vi "FDD COOLING SS Detector Self TRAINING Ver03.vi"() -> ()   [LabVIEW 2017]
uses:
  Control 1.ctl
  <vilib>/Utility/file.llb/Read Delimited Spreadsheet (string).vi
  <vilib>/Utility/file.llb/Write Delimited Spreadsheet (string).vi
  <vilib>/Analysis/NI_AALBase.lvlib
panel:
  out "SSD LOOP Counter":i32
  out "Loop2":bool
  out "Loop1":bool
  in  "Extract \nX&Y Data?":bool
  out "DONE":bool
  in  "PAUSE?":bool
  out "% Retained":dbl format="%.1f"
  out "SS Filtered\nArray Size":i32[](array[numeric])
  out "Pre-Processed Data\nArray Size":i32[](array[numeric])
  out "Time to Execute\nSCAN (millisecond)":dbl format="%.1f"
  in  "SAVE the Conditional\nand SSD Filtered Data?":bool
  out "Selected Data\nHeader Labels":string[](array[string])
  out "Data READ LOOP Counter":i32
  out "Data Filter LOOP Counter":i32
  in  "Tab Control":T1(tab)
  out "TOTAL FILES":i32
  out "Processing File # of":i32
  out "Current File":string
  in  "READ LIST\nto PROCESS":bool
  in  "END INDEX #":i32=10
  in  "START INDEX #":i32
  in  "Renumber Dependent\nVariable INDEX Array?":bool
  in  "Output File":path=path "C:/Vance/FDD Split System Project/FY2018 Univ of Connecticut DOE FDD Project/NIST RULE BASED CHART LABVIEW FDD CODE June 2018/SS-Example_RAW_Datafile.txt"
  out "X&Y Values - Selected String Array":string[][](array[string])
  in  "Dependent Variables\nY-Values Indices":i32[](array[numeric])=[161, 162, 163, 164, 165, 166, 167, 168, 169, 170, 171, 172, 173, 174, 175, 176, 177, 178, 179, 180, 181, 182, 183, 184, 185, 186, 187, 188, 189, 190, 191, 192, 193, 194, 195, 196, 197, 198, 199, 200, 201, 202, 203, 204, 205, 206, 207, 208, 209, 210, 211, 212, 213, 214, 215, 216, 217, 218, 219, 220, 221, 222, 223, 224, 225, 226, 227, 228, 229, 230, 231, 232, 233, 234, 235, 236, 237, 238, 239, 240, 241, 242, 243, 244, 245, 246, 247, 248, 249, 250, 251, 252, 253, 254, 255, 256, 257, 258, 259, 260, 261, 262, 263, 264, 265, 266, 267, 268, 269, 270, 271, 272, 273, 274, 275, 276, 277, 278, 279, 280, 281, 282, 283, 284, 285, 286, 287, 288, 289, 290, 291, 292, 293, 294, 295, 296, 297, 298, 299, 300, 301, 302, 303, 304, 305, 306, 307, 308, 309, 310, 311, 312, 313, 314, 315, 316, 317, 318, 319, 320, 321, 322, 323, 324, 325, 326, 327, 328, 329, 330, 331, 332, 333, 334, 335, 336, 337, 338, 339, 340, 341, 342, 343, 344, 345, 346, 347, 348, 349, 350, 351, 352, 353, 354, 355, 356, 357, 358, 359, 360, 361, 362, 363, 364, 365, 366, 367, 368, 369, 370, 371, 372, 373, 374, 375, 376, 377, 378, 379, 380, 381, 382, 383, 384, 385, 386, 387, 388, 389, 390, 391, 392, 393, 394, 395, 396, 397, 398, 399, 400, 401, 402, 403, 404, 405, 406, 407, 408, 409, 410, 411, 412, 413, 414, 415, 416, 417, 418, 419, 420]
  in  "Independent Variables\nX-Values Indices":i32[](array[numeric])=[160]
  out "Input File's Header Labels":string[](array[string])=["Count", "Date", "Time", "Elapsed_Sec", "RTD#1_C", "RTD#1_Ohm", "RTD#2_C", "RTD#2_Ohm", "IEQ_Date", "IEQ_Time", "IEQ_Sec", "1100", "1101", "1102", "1103", "1104", "1105", "1106", "1107", "1108", "1109", "1110", "1111", "1112", "1113", "1114", "1115", "1200", "1201", "1202", "1203", "1204", "1205", "1206", "1207", "1208", "1209", "1210", "1211", "1212", "1213", "1214", "1215", "1300", "1301", "1302", "1303", "1304", "1305", "1306", "1307", "1308", "1309", "1310", "1311", "1312", "1313", "1314", "1315"]
  in  "Input File":path=path "C:/Vance/FDD Split System Project/FY2018 Univ of Connecticut DOE FDD Project/NIST RULE BASED CHART LABVIEW FDD CODE June 2018/Example_RAW_Datafile.txt"
  in  "Append to File (T) or\nMake NEW FILE (F)?":bool=TRUE
  out "Write Output error out":errorcluster
  in  "Delete HEADER ROW?":bool=TRUE
  in  "SELECT Array of Tests":T3(array[cluster])=[{"Selected Data - COLUMN"=8.0, "Test Function"=0, "Test Value"=500.0, "Data Label"=""}, {"Selected Data - COLUMN"=4.0, "Test Function"=2, "Test Value"=5.0, "Data Label"=""}, {"Selected Data - COLUMN"=4.0, "Test Function"=0, "Test Value"=0.0, "Data Label"=""}, {"Selected Data - COLUMN"=208.0, "Test Function"=0, "Test Value"=100.0, "Data Label"=""}, {"Selected Data - COLUMN"=63.0, "Test Function"=0, "Test Value"=100.0, "Data Label"=""}]
  out "X&Y Values - Conditional Fiiltered Data":dbl[][](array[numeric])
  out "Pre-Processed Data\nArray Size 2":i32[](array[numeric])
  out "Array of Tests w/ Labels 3":T3(array[cluster])=[{"Selected Data - COLUMN"=8.0, "Test Function"=0, "Test Value"=500.0, "Data Label"="OD_Xitron_Watts"}, {"Selected Data - COLUMN"=7.0, "Test Function"=2, "Test Value"=20.0, "Data Label"="OD_Xitron_Amps"}, {"Selected Data - COLUMN"=4.0, "Test Function"=2, "Test Value"=3.0, "Data Label"="ID_Xitron_Amps"}, {"Selected Data - COLUMN"=4.0, "Test Function"=0, "Test Value"=0.3, "Data Label"="ID_Xitron_Amps"}, {"Selected Data - COLUMN"=193.0, "Test Function"=0, "Test Value"=0.25, "Data Label"="Unit ESP (in H2O)"}, {"Selected Data - COLUMN"=193.0, "Test Function"=2, "Test Value"=0.5, "Data Label"="Unit ESP (in H2O)"}]
  out "Array of Tests w/ Labels 2":T3(array[cluster])=[{"Selected Data - COLUMN"=8.0, "Test Function"=0, "Test Value"=500.0, "Data Label"="OD_Xitron_Watts"}, {"Selected Data - COLUMN"=7.0, "Test Function"=2, "Test Value"=20.0, "Data Label"="OD_Xitron_Amps"}, {"Selected Data - COLUMN"=4.0, "Test Function"=2, "Test Value"=3.0, "Data Label"="ID_Xitron_Amps"}, {"Selected Data - COLUMN"=4.0, "Test Function"=0, "Test Value"=0.3, "Data Label"="ID_Xitron_Amps"}, {"Selected Data - COLUMN"=193.0, "Test Function"=0, "Test Value"=0.25, "Data Label"="Unit ESP (in H2O)"}, {"Selected Data - COLUMN"=193.0, "Test Function"=2, "Test Value"=0.5, "Data Label"="Unit ESP (in H2O)"}]
  out "Array of Tests w/ Labels":T3(array[cluster])=[{"Selected Data - COLUMN"=8.0, "Test Function"=0, "Test Value"=500.0, "Data Label"="OD_Xitron_Watts"}, {"Selected Data - COLUMN"=7.0, "Test Function"=2, "Test Value"=20.0, "Data Label"="OD_Xitron_Amps"}, {"Selected Data - COLUMN"=4.0, "Test Function"=2, "Test Value"=3.0, "Data Label"="ID_Xitron_Amps"}, {"Selected Data - COLUMN"=4.0, "Test Function"=0, "Test Value"=0.3, "Data Label"="ID_Xitron_Amps"}, {"Selected Data - COLUMN"=193.0, "Test Function"=0, "Test Value"=0.25, "Data Label"="Unit ESP (in H2O)"}, {"Selected Data - COLUMN"=193.0, "Test Function"=2, "Test Value"=0.5, "Data Label"="Unit ESP (in H2O)"}]
  out "XY Graph2 Label 3":string
  out "XY Graph2 Label 2":string
  out "XY Graph2 Label":string
  out "XY Graph #1 4":cluster{dbl[], dbl[]}(graph)
  in  "XY Graph1\nX-Variable 4":i32=9
  in  "XY Graph1\nY-Variable 4":i32=194
  out "XY Graph #1 3":cluster{dbl[], dbl[]}(graph)
  out "XY Graph #1 2":cluster{dbl[], dbl[]}(graph)
  in  "XY Graph1\nX-Variable 2":i32=9
  in  "XY Graph1\nY-Variable 2":i32=181
  in  "XY Graph1\nX-Variable 3":i32=9
  in  "XY Graph1\nY-Variable 3":i32=82
  out "Mean Value Y2":dbl
  out "St. Dev. Y2":dbl
  out "Mean Value Y3":dbl
  out "St. Dev. Y3":dbl
  out "Mean Value Y4":dbl
  out "St. Dev. Y4":dbl
  out "XY Graph2 Label 6":string
  out "XY Graph #1 7":cluster{dbl[], dbl[]}(graph)
  in  "XY Graph1\nX-Variable 7":i32=9
  in  "XY Graph1\nY-Variable 7":i32=218
  out "XY Graph2 Label 5":string
  out "XY Graph #1 6":cluster{dbl[], dbl[]}(graph)
  in  "XY Graph1\nX-Variable 6":i32=9
  in  "XY Graph1\nY-Variable 6":i32=91
  out "XY Graph2 Label 4":string
  out "XY Graph #1 5":cluster{dbl[], dbl[]}(graph)
  in  "XY Graph1\nX-Variable 5":i32=9
  in  "XY Graph1\nY-Variable 5":i32=4
  out "Mean Value Y5":dbl
  out "St. Dev. Y5":dbl
  out "Mean Value Y6":dbl
  out "St. Dev. Y6":dbl
  out "Mean Value Y7":dbl
  out "St. Dev. Y7":dbl
  out "XY Graph2 Label 9":string
  out "XY Graph #1 10":cluster{dbl[], dbl[]}(graph)
  in  "XY Graph1\nX-Variable 10":i32=9
  in  "XY Graph1\nY-Variable 10":i32=257
  out "Mean Value Y7 4":dbl
  out "St. Dev. Y7 4":dbl
  out "XY Graph2 Label 8":string
  out "XY Graph #1 9":cluster{dbl[], dbl[]}(graph)
  in  "XY Graph1\nX-Variable 9":i32=9
  in  "XY Graph1\nY-Variable 9":i32=205
  out "Mean Value Y7 3":dbl
  out "St. Dev. Y7 3":dbl
  out "XY Graph2 Label 7":string
  out "XY Graph #1 8":cluster{dbl[], dbl[]}(graph)
  in  "XY Graph1\nX-Variable 8":i32=9
  in  "XY Graph1\nY-Variable 8":i32=222
  out "Mean Value Y7 2":dbl
  out "St. Dev. Y7 2":dbl
  out "Steady-State Monitoring Variables 4":T4(array[cluster])=[{"Y-Value for MW"=63.0, "Y MAX Std. Deviation"=1.4, "ABS Max SLOPE"=0.004655, "X-Value for MW"=9.0}, {"Y-Value for MW"=187.0, "Y MAX Std. Deviation"=0.5, "ABS Max SLOPE"=0.00096, "X-Value for MW"=9.0}, {"Y-Value for MW"=218.0, "Y MAX Std. Deviation"=1.0, "ABS Max SLOPE"=0.0065, "X-Value for MW"=9.0}, {"Y-Value for MW"=222.0, "Y MAX Std. Deviation"=0.75, "ABS Max SLOPE"=0.0065, "X-Value for MW"=9.0}, {"Y-Value for MW"=225.0, "Y MAX Std. Deviation"=0.4, "ABS Max SLOPE"=0.004, "X-Value for MW"=9.0}, {"Y-Value for MW"=246.0, "Y MAX Std. Deviation"=0.6, "ABS Max SLOPE"=0.005, "X-Value for MW"=9.0}, {"Y-Value for MW"=181.0, "Y MAX Std. Deviation"=0.1, "ABS Max SLOPE"=1000000000.0, "X-Value for MW"=9.0}, {"Y-Value for MW"=82.0, "Y MAX Std. Deviation"=0.1, "ABS Max SLOPE"=1000000000.0, "X-Value for MW"=9.0}, {"Y-Value for MW"=194.0, "Y MAX Std. Deviation"=0.1, "ABS Max SLOPE"=1000000000.0, "X-Value for MW"=9.0}] {"ABS Max SLOPE" step=0.05; "Y MAX Std. Deviation" step=0.05 format="%_6p"}
  out "Steady-State Monitoring Variables 3":T4(array[cluster])=[{"Y-Value for MW"=63.0, "Y MAX Std. Deviation"=1.4, "ABS Max SLOPE"=0.004655, "X-Value for MW"=9.0}, {"Y-Value for MW"=187.0, "Y MAX Std. Deviation"=0.5, "ABS Max SLOPE"=0.00096, "X-Value for MW"=9.0}, {"Y-Value for MW"=218.0, "Y MAX Std. Deviation"=1.0, "ABS Max SLOPE"=0.0065, "X-Value for MW"=9.0}, {"Y-Value for MW"=222.0, "Y MAX Std. Deviation"=0.75, "ABS Max SLOPE"=0.0065, "X-Value for MW"=9.0}, {"Y-Value for MW"=225.0, "Y MAX Std. Deviation"=0.4, "ABS Max SLOPE"=0.004, "X-Value for MW"=9.0}, {"Y-Value for MW"=246.0, "Y MAX Std. Deviation"=0.6, "ABS Max SLOPE"=0.005, "X-Value for MW"=9.0}, {"Y-Value for MW"=181.0, "Y MAX Std. Deviation"=0.1, "ABS Max SLOPE"=1000000000.0, "X-Value for MW"=9.0}, {"Y-Value for MW"=82.0, "Y MAX Std. Deviation"=0.1, "ABS Max SLOPE"=1000000000.0, "X-Value for MW"=9.0}, {"Y-Value for MW"=194.0, "Y MAX Std. Deviation"=0.1, "ABS Max SLOPE"=1000000000.0, "X-Value for MW"=9.0}] {"ABS Max SLOPE" step=0.05; "Y MAX Std. Deviation" step=0.05 format="%_6p"}
  out "Steady-State Monitoring Variables 2":T4(array[cluster])=[{"Y-Value for MW"=63.0, "Y MAX Std. Deviation"=1.4, "ABS Max SLOPE"=0.004655, "X-Value for MW"=9.0}, {"Y-Value for MW"=187.0, "Y MAX Std. Deviation"=0.5, "ABS Max SLOPE"=0.00096, "X-Value for MW"=9.0}, {"Y-Value for MW"=218.0, "Y MAX Std. Deviation"=1.0, "ABS Max SLOPE"=0.0065, "X-Value for MW"=9.0}, {"Y-Value for MW"=222.0, "Y MAX Std. Deviation"=0.75, "ABS Max SLOPE"=0.0065, "X-Value for MW"=9.0}, {"Y-Value for MW"=225.0, "Y MAX Std. Deviation"=0.4, "ABS Max SLOPE"=0.004, "X-Value for MW"=9.0}, {"Y-Value for MW"=246.0, "Y MAX Std. Deviation"=0.6, "ABS Max SLOPE"=0.005, "X-Value for MW"=9.0}, {"Y-Value for MW"=181.0, "Y MAX Std. Deviation"=0.1, "ABS Max SLOPE"=1000000000.0, "X-Value for MW"=9.0}, {"Y-Value for MW"=82.0, "Y MAX Std. Deviation"=0.1, "ABS Max SLOPE"=1000000000.0, "X-Value for MW"=9.0}, {"Y-Value for MW"=194.0, "Y MAX Std. Deviation"=0.1, "ABS Max SLOPE"=1000000000.0, "X-Value for MW"=9.0}] {"ABS Max SLOPE" step=0.05; "Y MAX Std. Deviation" step=0.05 format="%_6p"}
  in  "Steady-State Monitoring Variables":T4(array[cluster])=[{"Y-Value for MW"=63.0, "Y MAX Std. Deviation"=0.5, "ABS Max SLOPE"=0.1, "X-Value for MW"=9.0}, {"Y-Value for MW"=187.0, "Y MAX Std. Deviation"=0.5, "ABS Max SLOPE"=0.1, "X-Value for MW"=9.0}, {"Y-Value for MW"=218.0, "Y MAX Std. Deviation"=0.5, "ABS Max SLOPE"=0.1, "X-Value for MW"=9.0}, {"Y-Value for MW"=222.0, "Y MAX Std. Deviation"=0.5, "ABS Max SLOPE"=0.1, "X-Value for MW"=9.0}, {"Y-Value for MW"=225.0, "Y MAX Std. Deviation"=0.5, "ABS Max SLOPE"=0.1, "X-Value for MW"=9.0}, {"Y-Value for MW"=246.0, "Y MAX Std. Deviation"=0.4, "ABS Max SLOPE"=0.1, "X-Value for MW"=9.0}, {"Y-Value for MW"=181.0, "Y MAX Std. Deviation"=0.4, "ABS Max SLOPE"=0.1, "X-Value for MW"=9.0}, {"Y-Value for MW"=82.0, "Y MAX Std. Deviation"=0.4, "ABS Max SLOPE"=0.1, "X-Value for MW"=9.0}, {"Y-Value for MW"=194.0, "Y MAX Std. Deviation"=0.4, "ABS Max SLOPE"=0.1, "X-Value for MW"=9.0}] {"ABS Max SLOPE" step=0.05; "Y MAX Std. Deviation" step=0.05 format="%_6p"}
  in  "Moving \nWindow Size":i32=22
  out "X-Variable RANGE":dbl
  out "St. Dev. Y5 6":dbl
  out "Mean Value Y5 6":dbl
  out "XY Graph SS Filtered #1":cluster{dbl[], dbl[]}(graph)
  in  "XY Graph1\nX-Variable":i32=9
  in  "XY Graph1\nY-Variable":i32=63
  out "XY Graph1 Label":string
  out "XY Graph SS Filtered #2":cluster{dbl[], dbl[]}(graph)
  in  "XY Graph2\nX-Variable 5":i32=9
  in  "XY Graph2\nY-Variable 5":i32=218
  out "XY Graph1 Label 2":string
  out "Mean Value Y":dbl
  out "St. Dev. Y":dbl
  out "XY Graph1 Label 4":string
  in  "XY Graph2\nY-Variable 7":i32=225
  in  "XY Graph2\nX-Variable 7":i32=9
  out "XY Graph SS Filtered #4":cluster{dbl[], dbl[]}(graph)
  out "Mean Value Y5 3":dbl
  out "St. Dev. Y5 3":dbl
  out "XY Graph1 Label 3":string
  in  "XY Graph2\nY-Variable 6":i32=222
  in  "XY Graph2\nX-Variable 6":i32=9
  out "XY Graph SS Filtered #3":cluster{dbl[], dbl[]}(graph)
  out "Mean Value Y5 2":dbl
  out "St. Dev. Y5 2":dbl
  out "MW Calc ERROR OUT":errorcluster
  out "XY Graph1 Label 6":string
  in  "XY Graph2\nY-Variable 9":i32=184
  in  "XY Graph2\nX-Variable 9":i32=9
  out "XY Graph SS Filtered #6":cluster{dbl[], dbl[]}(graph)
  out "Mean Value Y5 5":dbl
  out "St. Dev. Y5 5":dbl
  out "XY Graph1 Label 5":string
  in  "XY Graph2\nY-Variable 8":i32=246
  in  "XY Graph2\nX-Variable 8":i32=9
  out "XY Graph SS Filtered #5":cluster{dbl[], dbl[]}(graph)
  out "Mean Value Y5 4":dbl
  out "St. Dev. Y5 4":dbl
  out "DONE 3":bool
  out "DONE 4":bool
  out "DONE 2":bool
  # "Grab and Filter Data"
  # "Rows"
  # "Columns"
  # "Apply Conditional Filters to the Selected Data"
  # "ROWS"
  # "COLS"
  # "Conditional Filtered Data PLOTS"
  # "Conditional Filtered Data PLOTS"
  # "Conditional & SSD Filtered Data PLOTS"
  # "Display all the SS Monitoring Variables on ONE SCREEN"
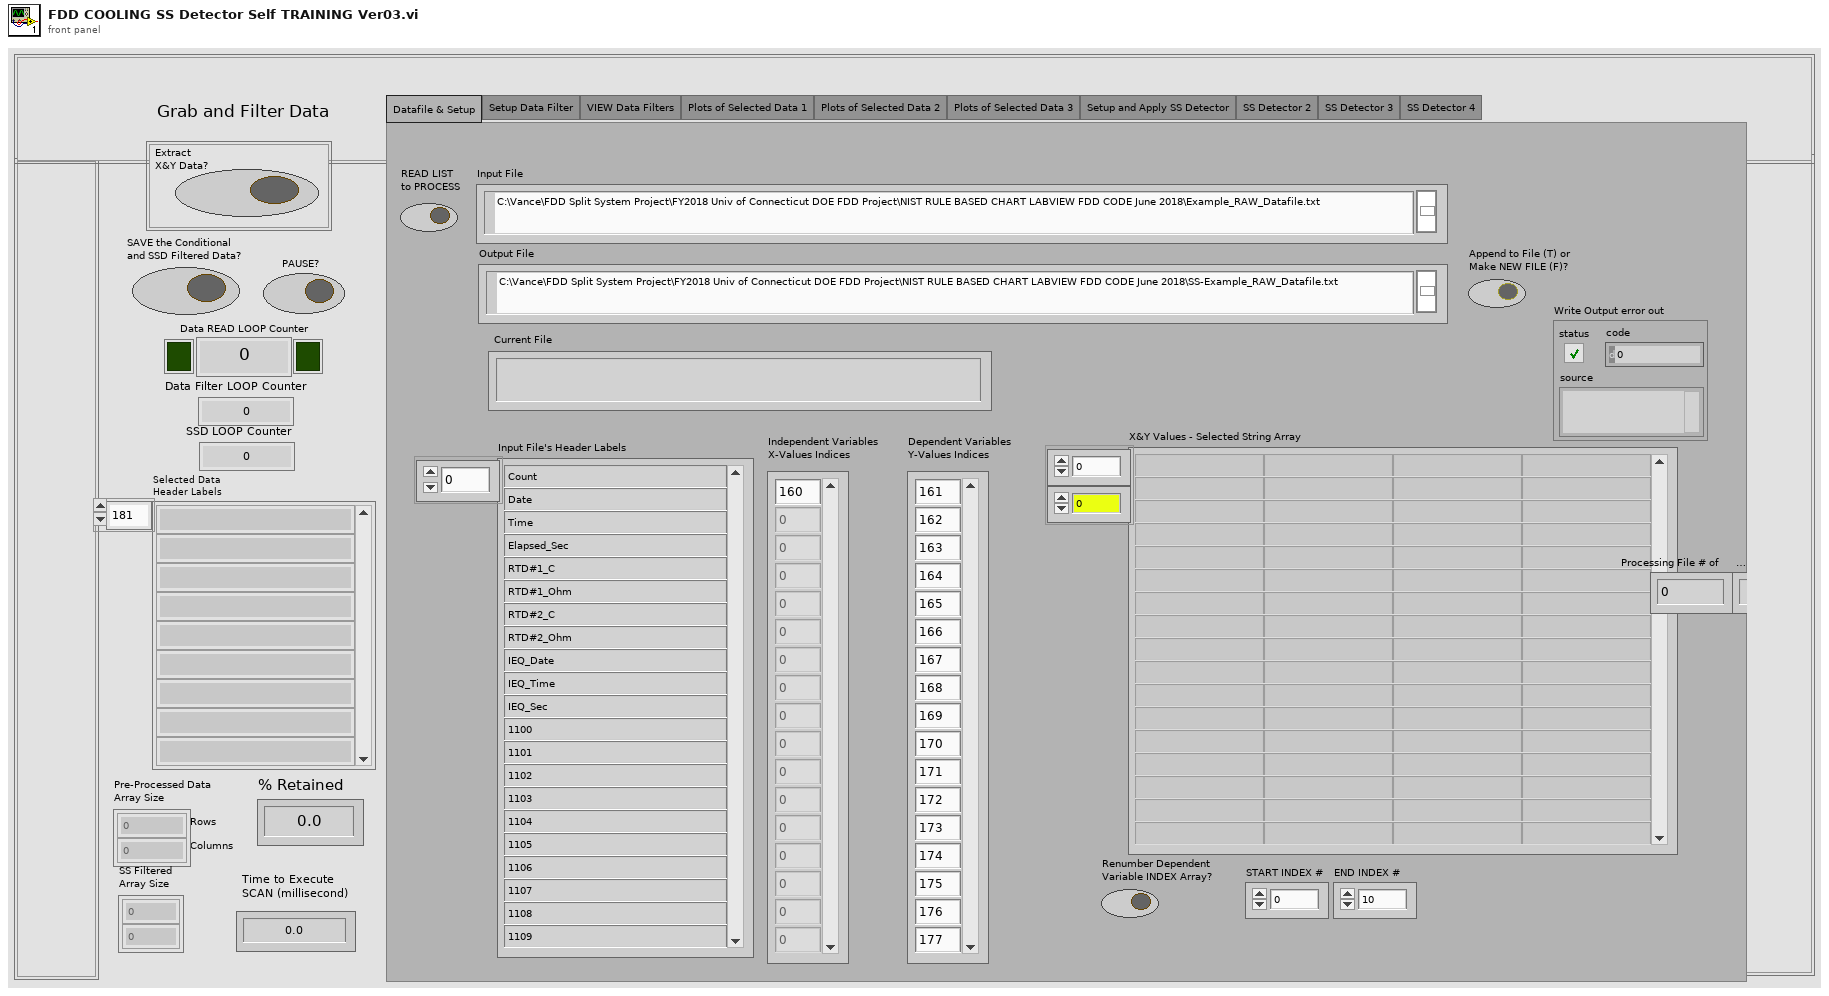
[diagram p1: front panel]
types:
  T1 = enum32{"Datafile & Setup", "Setup Data Filter", "VIEW Data Filters", "Plots of Selected Data 1", "Plots of Selected Data 2", "Plots of Selected Data 3", "Setup and Apply SS Detector", "SS Detector 2", "SS Detector 3", "SS Detector 4"}
  T2 = typedef "Control 1.ctl" = i32
  T3 = cluster{"Selected Data - COLUMN":dbl, "Test Function":T2, "Test Value":dbl, "Data Label":string}[]
  T4 = cluster{"Y-Value for MW":dbl, "Y MAX Std. Deviation":dbl, "ABS Max SLOPE":dbl, "X-Value for MW":dbl}[]
  T5 = cluster{"Selected Data - COLUMN":dbl, "Test Function":T2, "Test Value":dbl, "Data Label":string}
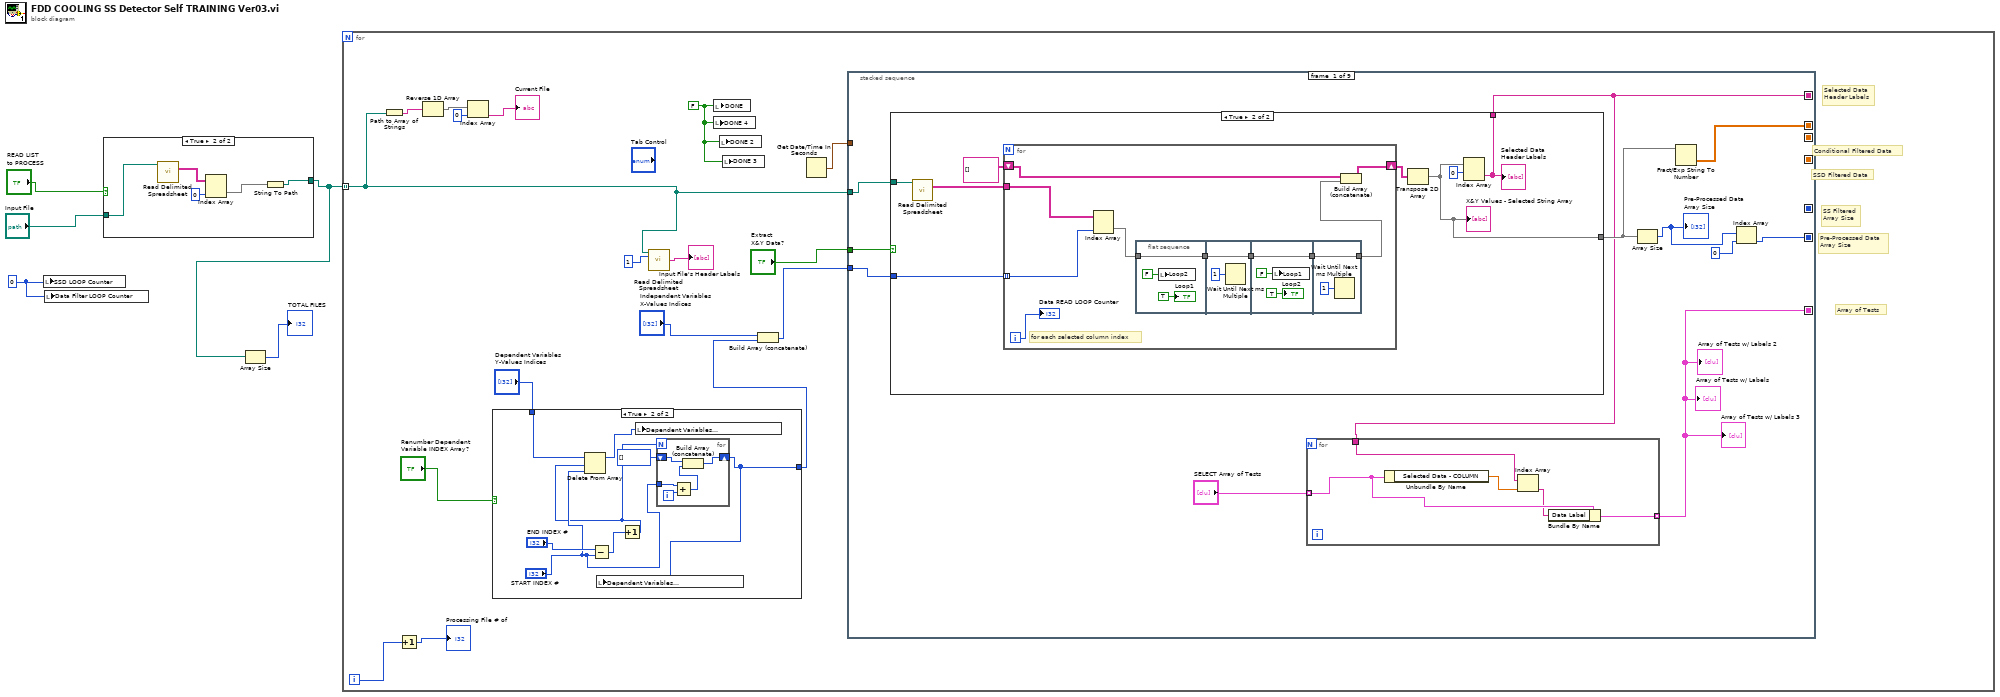
[diagram p0: block diagram]
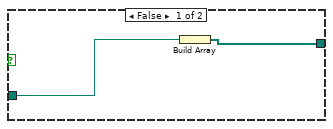
[diagram p2: hidden frame]
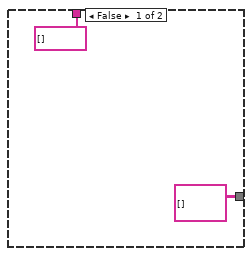
[diagram p4: hidden frame]
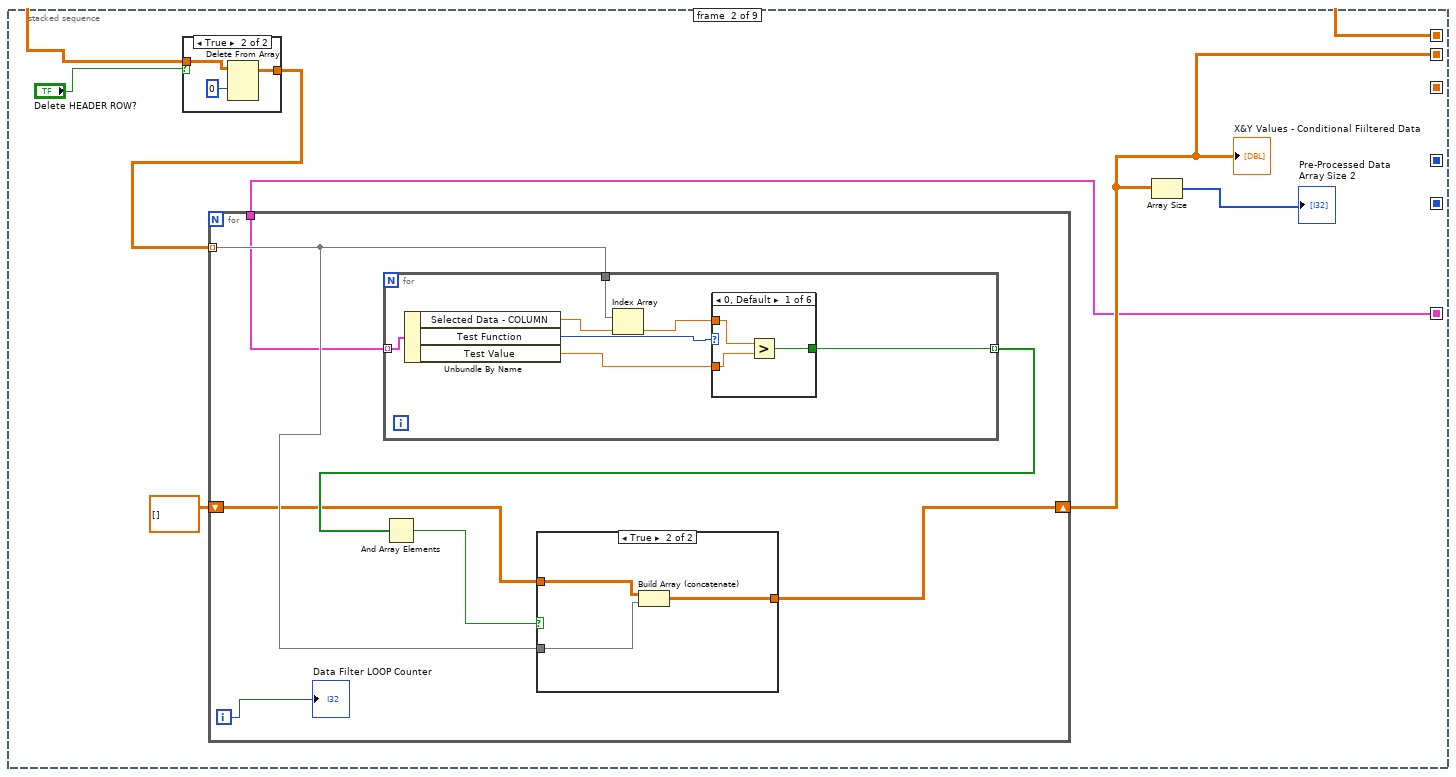
[diagram p5: hidden frame]
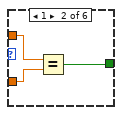
[diagram p8: hidden frame]
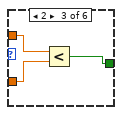
[diagram p9: hidden frame]
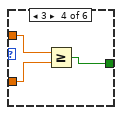
[diagram p10: hidden frame]
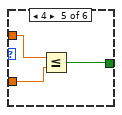
[diagram p11: hidden frame]
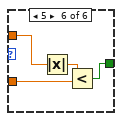
[diagram p12: hidden frame]
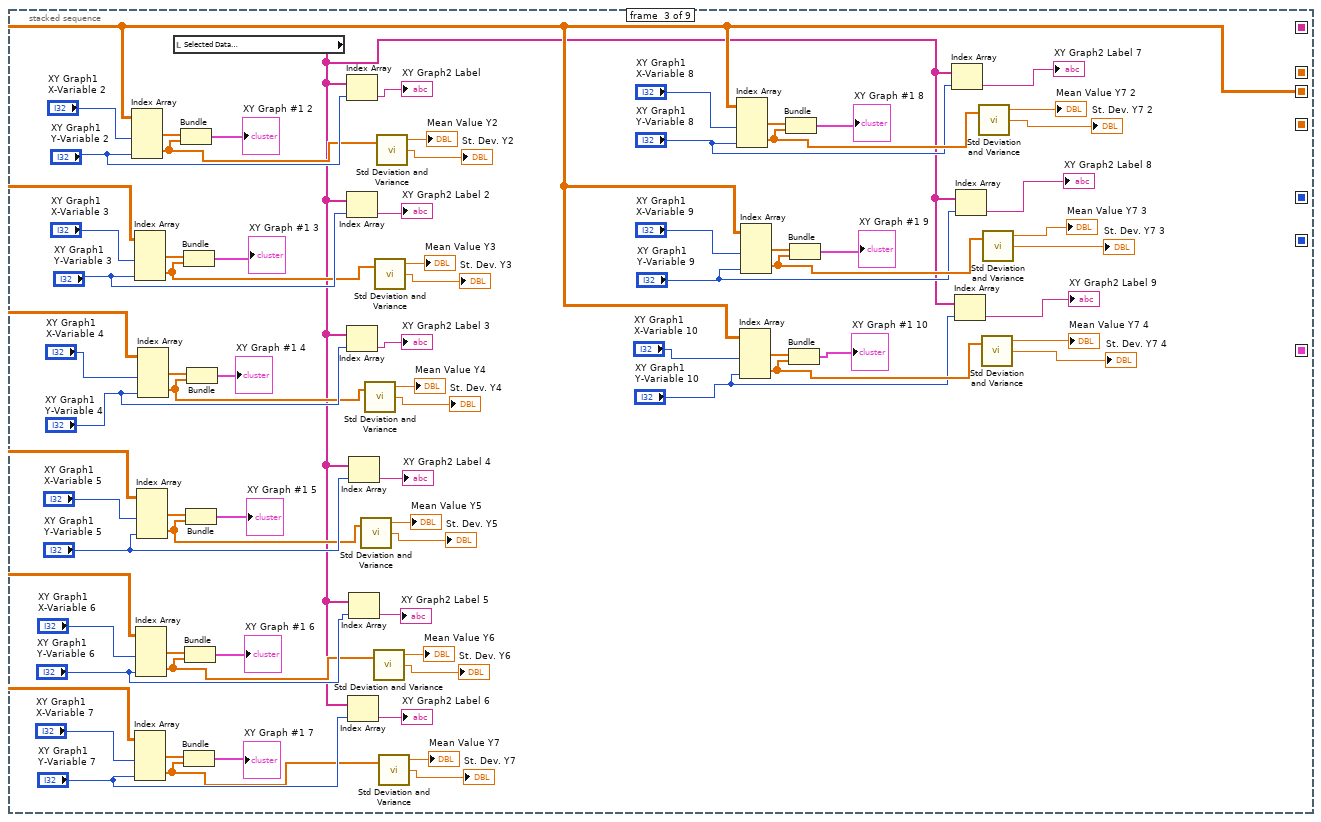
[diagram p13: hidden frame]
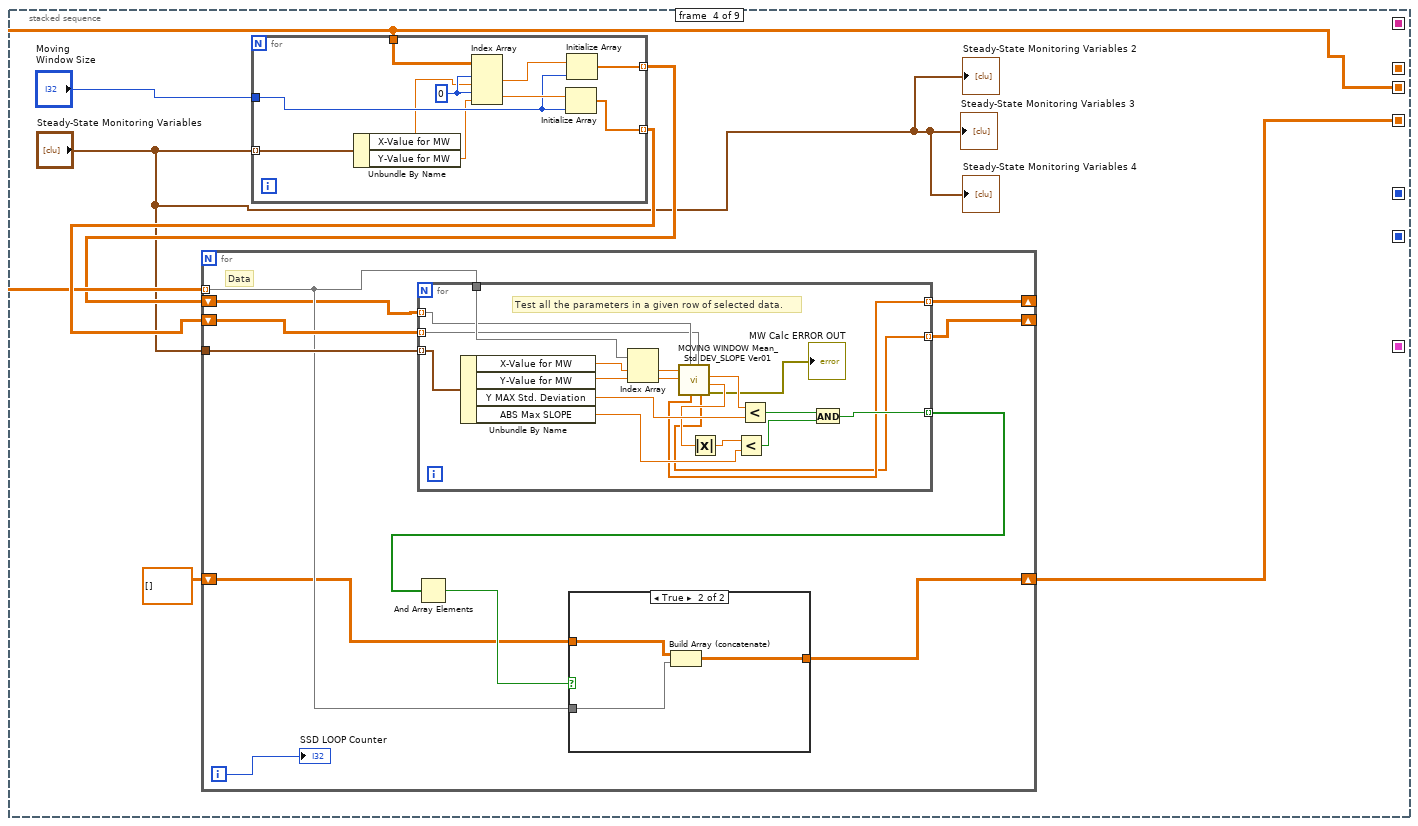
[diagram p14: hidden frame]
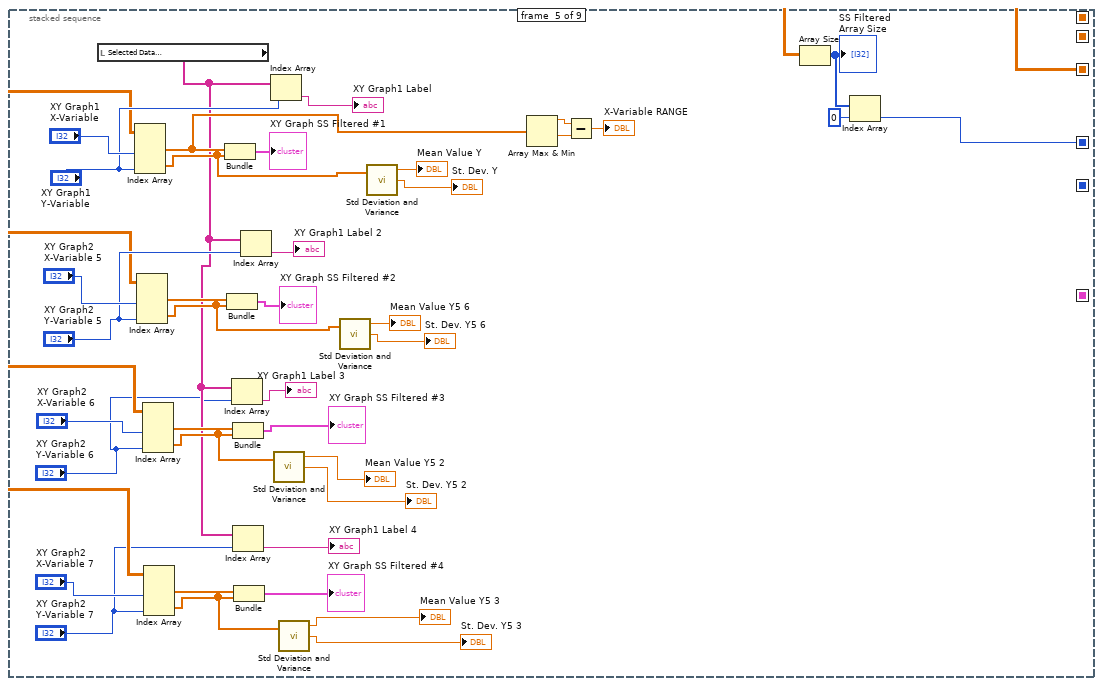
[diagram p16: hidden frame]
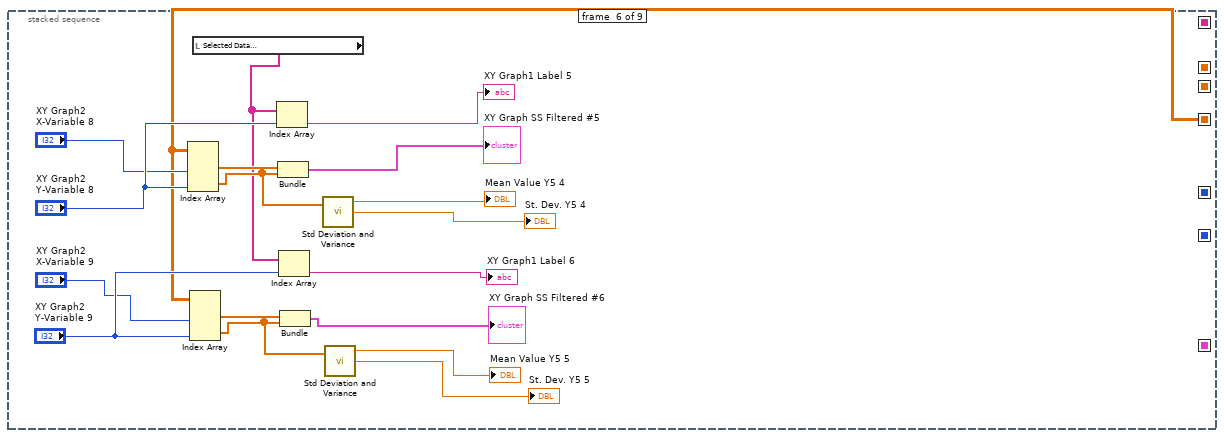
[diagram p17: hidden frame]
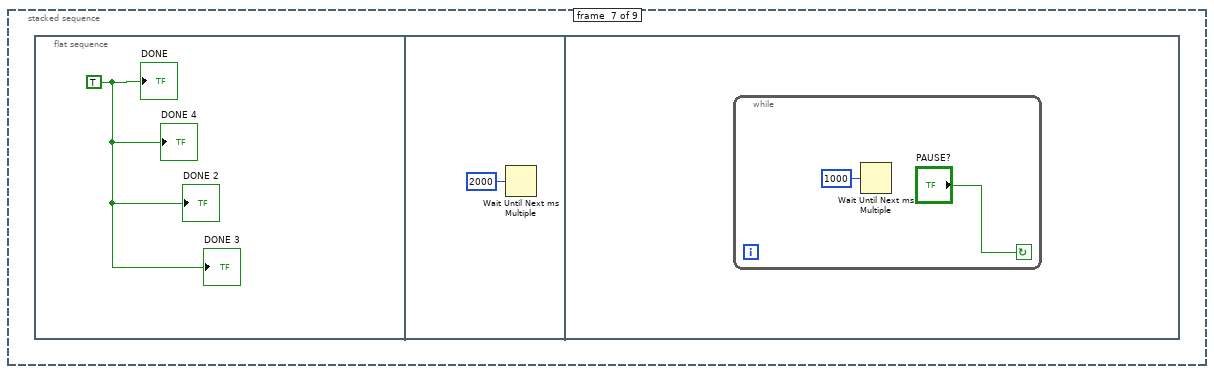
[diagram p18: hidden frame]
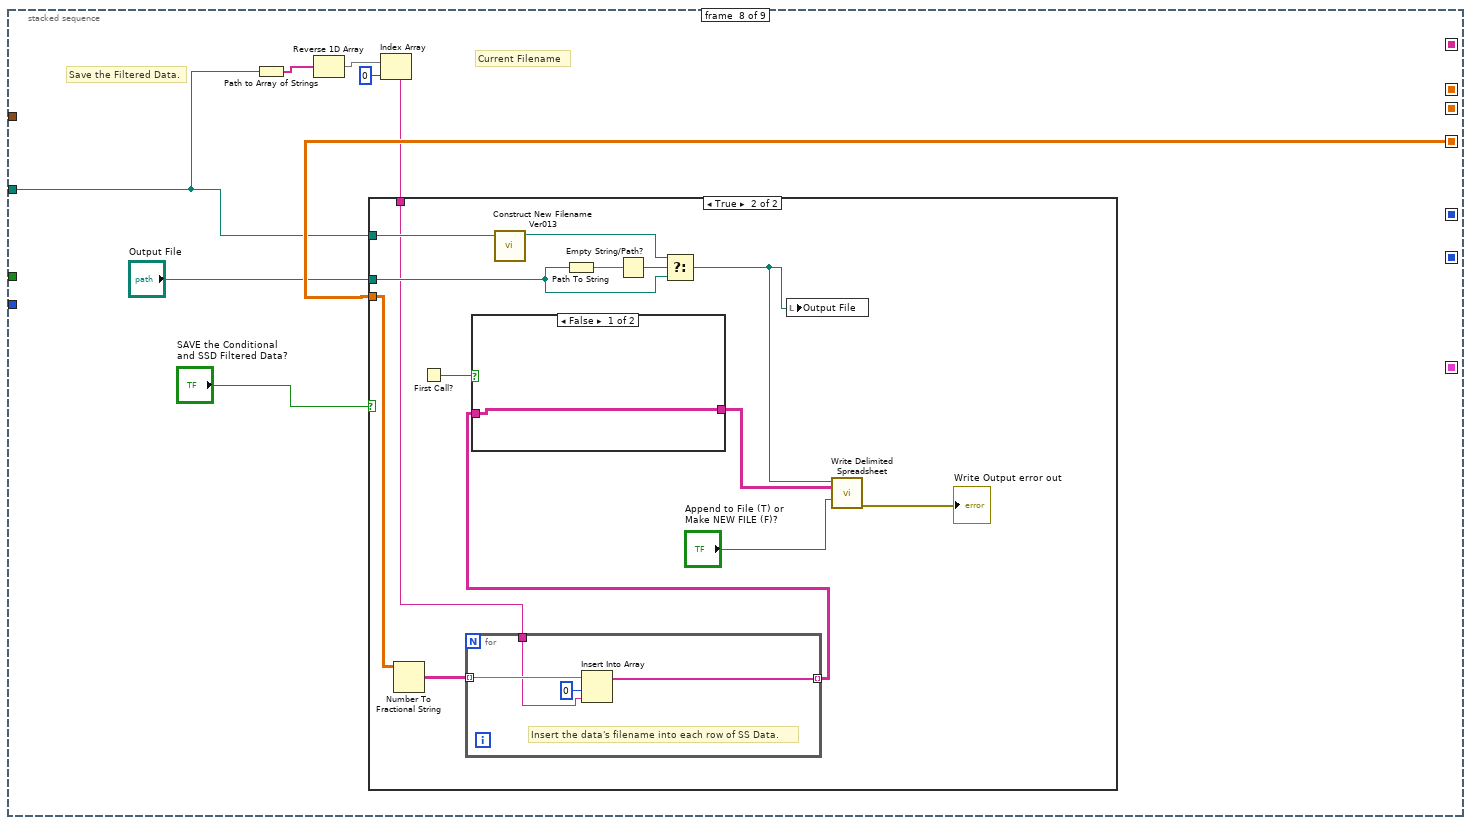
[diagram p19: hidden frame]
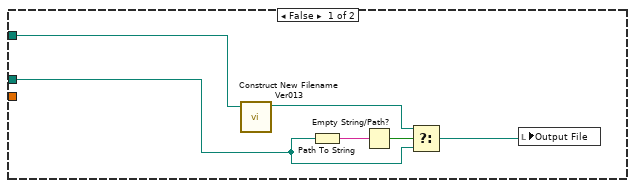
[diagram p20: hidden frame]
diagram:
  w1 = 0 ("SSD LOOP Counter")
  n1 = local write "SSD LOOP Counter"(w1) -> ()
  n2 = local write "Data Filter LOOP Counter"(w1) -> ()
  n3 = case shown="True" "READ LIST\nto PROCESS" {
    tunnel: "Input File" -> [w7 w12]
    tunnel: [w6 w8] -> w3
    frame False {
      n4 = Build Array(w7) -> (w6:path[])
    }
    frame True {
      n5 = call-poly <vilib>:"Read Delimited Spreadsheet.vi"("file path (dialog if empty)"=w12) -> ("all rows"=w11:string[][])  [unwired: 9 in, 5 out]
      n6 = Index Array(array=w11, index (col)=0 ("disabled index (col)")) -> (element=w9:string[])  [unwired: 1 in]
      n7 = String To Path(string=w9) -> (path=w8:path[])
    }
  }
  n8 = Array Size(array=w3) -> (size(s)=→"TOTAL FILES":i32)
  n9 = for {
    tunnel: w3 -> [w17] mode=indexing
    i -> [w15]
    w21 = FALSE ("DONE")
    # "Array of Tests"
    # "Selected Data\nHeader Labels"
    # "SS Filtered\nArray Size"
    # "Pre-Processed Data\nArray Size"
    # "Conditional Filtered Data"
    # "SSD Filtered Data"
    n10 = Path to Array of Strings(0:w17) -> (2:w20:string[])  [unwired: 1 out]
    n11 = Increment(x=w15) -> (x+1=→"Processing File # of":i32)
    n12 = Reverse 1D Array(array=w20) -> (reversed array=w19:string[])
    n13 = Index Array(array=w19, index=0) -> (element=→"Current File":string)
    n14 = case shown="True" "Renumber Dependent\nVariable INDEX Array?" {
      tunnel: "Dependent Variables\nY-Values Indices" -> [w30 w38]
      tunnel: [w30 w31] -> w23
      frame False {
      }
      frame True {
        n15 = Subtract(x="END INDEX #", y="START INDEX #") -> (x-y=w36:i32)
        n16 = Increment(x=w36) -> (x+1=w33:i32)
        n17 = Delete From Array(array=w38, length=w33, index="START INDEX #") -> (array with subset deleted=w34:i32[])  [unwired: 1 out]
        n18 = local write "Dependent Variables\nY-Values Indices"(w34) -> ()
        n19 = for {
          N: w33 -> [_]
          tunnel: "START INDEX #" -> [w42]
          shift-right: [w40] -> w31
          shift-left: i32[] [] -> [w39]
          i -> [w43]
          n20 = Add(x=w42, y=w43) -> (x+y=w41:i32)
          n21 = Build Array (concatenate)(w39, w41) -> (w40:i32[])
        }
        n22 = local write "Dependent Variables\nY-Values Indices"(w31) -> ()
      }
    }
    n23 = call-poly <vilib>:"Read Delimited Spreadsheet.vi"("file path (dialog if empty)"=w17, "number of rows (all:-1)"=1) -> ("first row"=→"Input File's Header Labels":string[])  [unwired: 8 in, 5 out]
    n24 = local write "DONE 4"(w21) -> ()
    n25 = local write "DONE"(w21) -> ()
    n26 = local write "DONE 2"(w21) -> ()
    n27 = local write "DONE 3"(w21) -> ()
    n28 = Build Array (concatenate)("Independent Variables\nX-Values Indices", w23) -> (w27:i32[])
    n29 = Get Date/Time In Seconds() -> (seconds since 1Jan1904=w25:timestamp)
    n30 = stacked-sequence {
      seq-local: [w54 _ _ _ _ _ _ _ _] -> [_ w93 _ _ _ _ _ _ _]
      seq-local: [_ w94 _ _ _ _ _ _ _] -> [_ _ w139 w216 _ _ _ _ _]
      seq-local: [_ _ _ w214 _ _ _ _ _] -> [_ _ _ _ w274 w307 _ w331 _]
      seq-local: [_ _ _ _ w264 _ _ _ _] -> [_ _ _ _ _ _ _ _ w367]
      seq-local: [w48 _ _ _ _ _ _ _ _] -> [_ _ _ _ _ _ _ _ w365]
      seq-local: [w45 _ _ _ _ _ _ _ _] -> [_ _ _ _ _ _ _ _ _]
      seq-local: [w44 _ _ _ _ _ _ _ _] -> [_ w90 _ _ _ _ _ _ _]
      tunnel: w17 -> [w49 _ _ _ _ _ _ w329 _]
      tunnel: w27 -> [w52 _ _ _ _ _ _ _ _]
      tunnel: "Extract \nX&Y Data?" -> [w51 _ _ _ _ _ _ _ _]
      tunnel: w25 -> [_ _ _ _ _ _ _ _ w375]
      frame #0 {
        n31 = case shown="True" w51 {
          tunnel: w52 -> [_ w69]
          tunnel: [string[][] [] w63] -> w50
          tunnel: w49 -> [_ w66]
          tunnel: [string[] [] w62] -> w45
          frame False {
          }
          frame True {
            n32 = call-poly <vilib>:"Read Delimited Spreadsheet.vi"("file path (dialog if empty)"=w66) -> ("all rows"=w65:string[][])  [unwired: 9 in, 5 out]
            n33 = for {
              tunnel: w69 -> [w78] mode=indexing
              tunnel: w65 -> [w79]
              shift-right: [w77] -> w64
              shift-left: string[][] [] -> [w76]
              i -> [w75]
              # "for each selected column index"
              n34 = Index Array(array=w79, index (col)=w78) -> (element=w73:string[])  [unwired: 1 in]
              n35 = flat-sequence {
                tunnel: [w80] -> w74
                tunnel: w73 -> [w80]
                tunnel: w74 -> [w83]
                tunnel: [w83] -> w72
                tunnel: w72 -> [w85]
                tunnel: [w85] -> w71
                tunnel: w71 -> [w88]
                tunnel: [w88] -> w70
                frame #0 {
                  n36 = local write "Loop2"(FALSE ("Loop2")) -> ()
                  "Loop1" <- TRUE ("Loop1")
                }
                frame #1 {
                  n37 = Wait Until Next ms Multiple(millisecond multiple=u32 1) -> ()  [unwired: 1 out]
                }
                frame #2 {
                  n38 = local write "Loop1"(FALSE ("Loop1")) -> ()
                  "Loop2" <- TRUE ("Loop2")
                }
                frame #3 {
                  n39 = Wait Until Next ms Multiple(millisecond multiple=u32 1) -> ()  [unwired: 1 out]
                }
              }
              n40 = Build Array (concatenate)(w76, w70) -> (w77:string[][])
              "Data READ LOOP Counter" <- w75
            }
            n41 = Transpose 2D Array(2D array=w64) -> (transposed array=w63:string[][])
            "X&Y Values - Selected String Array" <- w63
            n42 = Index Array(array=w63, index (row)=0) -> (element=w62:string[])  [unwired: 1 in]
            "Selected Data\nHeader Labels" <- w62
          }
        }
        n43 = for {
          tunnel: "SELECT Array of Tests" -> [w57] mode=indexing
          tunnel: w45 -> [w59]
          tunnel: [w55] -> w44 mode=indexing
          n44 = Unbundle By Name(w57) -> ("Selected Data - COLUMN"=w58:dbl)
          n45 = Index Array(array=w59, index=w58) -> (element=w56:string)
          n46 = Bundle By Name(cluster=w57, "Data Label"=w56) -> (w55:T5)
        }
        "Array of Tests w/ Labels" <- w44
        "Array of Tests w/ Labels 2" <- w44
        "Array of Tests w/ Labels 3" <- w44
        n47 = Array Size(array=w50) -> (size(s)=w53:i32[])
        "Pre-Processed Data\nArray Size" <- w53
        n48 = Fract/Exp String To Number(string=w50) -> (number=w54:dbl[][])  [unwired: 3 in, 1 out]
        n49 = Index Array(array=w53, index=0) -> (element=w48:i32)
      }
      frame #1 {
        n50 = case shown="True" "Delete HEADER ROW?" {
          tunnel: w93 -> [w97 w100]
          tunnel: [w97 w98] -> w91
          frame False {
          }
          frame True {
            n51 = Delete From Array(array=w100, index (row)=0) -> (array with subset deleted=w98:dbl[][])  [unwired: 2 in, 1 out]
          }
        }
        n52 = for {
          tunnel: w91 -> [w105] mode=indexing
          shift-right: [w104] -> w94
          shift-left: dbl[][] [] -> [w103]
          tunnel: w90 -> [w101]
          i -> [w102]
          n53 = for {
            tunnel: w101 -> [w118] mode=indexing
            tunnel: w105 -> [w117]
            tunnel: [w112] -> w107 mode=indexing
            n54 = Unbundle By Name "Unbundle By Name"(w118) -> ("Selected Data - COLUMN"=w116:dbl, "Test Function"=w115:T2, "Test Value"=w113:dbl)
            n55 = Index Array(array=w117, index=w116) -> (element=w114:dbl)
            n56 = case shown="0, Default" w115 {
              tunnel: w114 -> [w121 w124 w127 w130 w133 w137]
              tunnel: w113 -> [w120 w123 w126 w129 w132 w135]
              tunnel: [w119 w122 w125 w128 w131 w134] -> w112
              frame 0, Default {
                n57 = Greater?(x=w121, y=w120) -> (0:w119:bool)
              }
              frame 1 {
                n58 = Equal?(x=w124, y=w123) -> (x = y?=w122:bool)
              }
              frame 2 {
                n59 = Less?(x=w127, y=w126) -> (x < y?=w125:bool)
              }
              frame 3 {
                n60 = Greater Or Equal?(x=w130, y=w129) -> (x >= y?=w128:bool)
              }
              frame 4 {
                n61 = Less Or Equal?(x=w133, y=w132) -> (x <= y?=w131:bool)
              }
              frame 5 {
                n62 = Absolute Value(x=w137) -> (abs(x)=w136:dbl)
                n63 = Less?(x=w136, y=w135) -> (x < y?=w134:bool)
              }
            }
          }
          n64 = And Array Elements(Boolean array=w107) -> (logical AND=w106:bool)
          n65 = case shown="True" w106 {
            tunnel: w105 -> [_ w111]
            tunnel: [w108 w110] -> w104
            tunnel: w103 -> [w108 w109]
            frame False {
            }
            frame True {
              n66 = Build Array (concatenate)(w109, w111) -> (w110:dbl[][])
            }
          }
          "Data Filter LOOP Counter" <- w102
        }
        "X&Y Values - Conditional Fiiltered Data" <- w94
        n67 = Array Size(array=w94) -> (size(s)=→"Pre-Processed Data\nArray Size 2":i32[])
      }
      frame #2 {
        n68 = Index Array(array=w139, index (col) #1="XY Graph1\nX-Variable 2", index (col) #2="XY Graph1\nY-Variable 2") -> (element #1=w164:dbl[], element #2=w180:dbl[])  [unwired: 2 in]
        n69 = Index Array(array=w139, index (col) #1="XY Graph1\nX-Variable 3", index (col) #2="XY Graph1\nY-Variable 3") -> (element #1=w208:dbl[], element #2=w177:dbl[])  [unwired: 2 in]
        n70 = Index Array(array=w139, index (col) #1="XY Graph1\nX-Variable 7", index (col) #2="XY Graph1\nY-Variable 7") -> (element #1=w191:dbl[], element #2=w165:dbl[])  [unwired: 2 in]
        n71 = Index Array(array=w139, index (col) #1="XY Graph1\nX-Variable 6", index (col) #2="XY Graph1\nY-Variable 6") -> (element #1=w192:dbl[], element #2=w168:dbl[])  [unwired: 2 in]
        n72 = Index Array(array=w139, index (col) #1="XY Graph1\nX-Variable 5", index (col) #2="XY Graph1\nY-Variable 5") -> (element #1=w197:dbl[], element #2=w171:dbl[])  [unwired: 2 in]
        n73 = Index Array(array=w139, index (col) #1="XY Graph1\nX-Variable 4", index (col) #2="XY Graph1\nY-Variable 4") -> (element #1=w207:dbl[], element #2=w174:dbl[])  [unwired: 2 in]
        n74 = local read "Selected Data\nHeader Labels"() -> (w138:string[])
        n75 = Bundle(w164, w180) -> (→"XY Graph #1 2":cluster{dbl[], dbl[]})  [unwired: 1 in]
        n76 = Bundle(w208, w177) -> (→"XY Graph #1 3":cluster{dbl[], dbl[]})  [unwired: 1 in]
        n77 = Bundle(w191, w165) -> (→"XY Graph #1 7":cluster{dbl[], dbl[]})  [unwired: 1 in]
        n78 = Bundle(w192, w168) -> (→"XY Graph #1 6":cluster{dbl[], dbl[]})  [unwired: 1 in]
        n79 = Bundle(w197, w171) -> (→"XY Graph #1 5":cluster{dbl[], dbl[]})  [unwired: 1 in]
        n80 = Bundle(w207, w174) -> (→"XY Graph #1 4":cluster{dbl[], dbl[]})  [unwired: 1 in]
        n81 = Index Array(array=w138, index="XY Graph1\nY-Variable 2") -> (element=→"XY Graph2 Label":string)
        n82 = Index Array(array=w138, index="XY Graph1\nY-Variable 3") -> (element=→"XY Graph2 Label 2":string)
        n83 = Index Array(array=w138, index="XY Graph1\nY-Variable 4") -> (element=→"XY Graph2 Label 3":string)
        n84 = Index Array(array=w138, index="XY Graph1\nY-Variable 7") -> (element=→"XY Graph2 Label 6":string)
        n85 = Index Array(array=w138, index="XY Graph1\nY-Variable 5") -> (element=→"XY Graph2 Label 4":string)
        n86 = Index Array(array=w138, index="XY Graph1\nY-Variable 6") -> (element=→"XY Graph2 Label 5":string)
        n87 = call <vilib>:"Std Deviation and Variance.vi"("X"=w171) -> ("mean"=→"Mean Value Y5":dbl, "standard deviation"=→"St. Dev. Y5":dbl)  [unwired: 1 in, 1 out]
        n88 = call <vilib>:"Std Deviation and Variance.vi"("X"=w174) -> ("mean"=→"Mean Value Y4":dbl, "standard deviation"=→"St. Dev. Y4":dbl)  [unwired: 1 in, 1 out]
        n89 = call <vilib>:"Std Deviation and Variance.vi"("X"=w168) -> ("mean"=→"Mean Value Y6":dbl, "standard deviation"=→"St. Dev. Y6":dbl)  [unwired: 1 in, 1 out]
        n90 = call <vilib>:"Std Deviation and Variance.vi"("X"=w177) -> ("mean"=→"Mean Value Y3":dbl, "standard deviation"=→"St. Dev. Y3":dbl)  [unwired: 1 in, 1 out]
        n91 = call <vilib>:"Std Deviation and Variance.vi"("X"=w180) -> ("mean"=→"Mean Value Y2":dbl, "standard deviation"=→"St. Dev. Y2":dbl)  [unwired: 1 in, 1 out]
        n92 = call <vilib>:"Std Deviation and Variance.vi"("X"=w165) -> ("mean"=→"Mean Value Y7":dbl, "standard deviation"=→"St. Dev. Y7":dbl)  [unwired: 1 in, 1 out]
        n93 = Index Array(array=w139, index (col) #1="XY Graph1\nX-Variable 8", index (col) #2="XY Graph1\nY-Variable 8") -> (element #1=w162:dbl[], element #2=w163:dbl[])  [unwired: 2 in]
        n94 = Index Array(array=w139, index (col) #1="XY Graph1\nX-Variable 10", index (col) #2="XY Graph1\nY-Variable 10") -> (element #1=w146:dbl[], element #2=w147:dbl[])  [unwired: 2 in]
        n95 = Index Array(array=w139, index (col) #1="XY Graph1\nX-Variable 9", index (col) #2="XY Graph1\nY-Variable 9") -> (element #1=w154:dbl[], element #2=w155:dbl[])  [unwired: 2 in]
        n96 = Bundle(w162, w163) -> (→"XY Graph #1 8":cluster{dbl[], dbl[]})  [unwired: 1 in]
        n97 = Bundle(w146, w147) -> (→"XY Graph #1 10":cluster{dbl[], dbl[]})  [unwired: 1 in]
        n98 = Bundle(w154, w155) -> (→"XY Graph #1 9":cluster{dbl[], dbl[]})  [unwired: 1 in]
        n99 = Index Array(array=w138, index="XY Graph1\nY-Variable 8") -> (element=→"XY Graph2 Label 7":string)
        n100 = Index Array(array=w138, index="XY Graph1\nY-Variable 10") -> (element=→"XY Graph2 Label 9":string)
        n101 = Index Array(array=w138, index="XY Graph1\nY-Variable 9") -> (element=→"XY Graph2 Label 8":string)
        n102 = call <vilib>:"Std Deviation and Variance.vi"("X"=w163) -> ("mean"=→"Mean Value Y7 2":dbl, "standard deviation"=→"St. Dev. Y7 2":dbl)  [unwired: 1 in, 1 out]
        n103 = call <vilib>:"Std Deviation and Variance.vi"("X"=w147) -> ("mean"=→"Mean Value Y7 4":dbl, "standard deviation"=→"St. Dev. Y7 4":dbl)  [unwired: 1 in, 1 out]
        n104 = call <vilib>:"Std Deviation and Variance.vi"("X"=w155) -> ("mean"=→"Mean Value Y7 3":dbl, "standard deviation"=→"St. Dev. Y7 3":dbl)  [unwired: 1 in, 1 out]
      }
      frame #3 {
        n105 = for {
          tunnel: "Steady-State Monitoring Variables" -> [w262] mode=indexing
          tunnel: "Moving \nWindow Size" -> [w257]
          tunnel: [w261] -> w217 mode=indexing
          tunnel: w216 -> [w259]
          tunnel: [w255] -> w213 mode=indexing
          w258 = 0 ("disabled index (row)")
          n106 = Unbundle By Name(w262) -> ("X-Value for MW"=w254:dbl, "Y-Value for MW"=w253:dbl)
          n107 = Index Array "Index Array"(array=w259, index (row) #1=w258, index (col) #1=w254, index (row) #2=w258, index (col) #2=w253) -> (element #1=w256:dbl, element #2=w260:dbl)
          n108 = Initialize Array(w260, w257) -> (w261:dbl[])
          n109 = Initialize Array "Initialize Array"(w256, w257) -> (w255:dbl[])
        }
        n110 = for {
          tunnel: w216 -> [w224] mode=indexing
          tunnel: "Steady-State Monitoring Variables" -> [w229]
          shift-right: [w227] -> _
          shift-left: w217 -> [w228]
          shift-right: [w222] -> w214
          shift-left: dbl[][] [] -> [w223]
          shift-right: [w220] -> _
          shift-left: w213 -> [w221]
          i -> [w219]
          # "Data"
          n111 = for {
            tunnel: w228 -> [w237] mode=indexing
            tunnel: w229 -> [w252] mode=indexing
            tunnel: w224 -> [w243]
            tunnel: [w244] -> w225 mode=indexing
            tunnel: [w235] -> w227 mode=indexing
            tunnel: w221 -> [w238] mode=indexing
            tunnel: [w236] -> w220 mode=indexing
            # "Test all the parameters in a given row of selected data."
            n112 = Unbundle By Name(w252) -> ("X-Value for MW"=w242:dbl, "Y-Value for MW"=w241:dbl, "Y MAX Std. Deviation"=w251:dbl, "ABS Max SLOPE"=w247:dbl)
            n113 = Index Array(array=w243, index #1=w242, index #2=w241) -> (element #1=w240:dbl, element #2=w239:dbl)
            n114 = call "MOVING WINDOW Mean_Std DEV_SLOPE Ver01.vi"("OLD Moving Window Values"=w237, "OLD Time or Scan# Values\n(X-Values for SLOPE Calc)"=w238, "NEW Moving Window \nArray ELEMENT"=w239, "NEW Moving Window \nTime Array ELEMENT"=w240) -> ("error out"=→"MW Calc ERROR OUT":errorcluster, "MW SLOPE"=w248:dbl, "MW Std. Dev."=w250:dbl, "NEW Moving Window Values"=w235:dbl[], "NEW Time or Scan# Values"=w236:dbl[])  [unwired: 2 in, 1 out]
            n115 = Absolute Value(x=w248) -> (abs(x)=w249:dbl)
            n116 = Less?(x=w249, y=w247) -> (x < y?=w246:bool)
            n117 = Less?(x=w250, y=w251) -> (x < y?=w245:bool)
            n118 = And(x=w245, y=w246) -> (x .and. y?=w244:bool)
          }
          n119 = And Array Elements(Boolean array=w225) -> (logical AND=w226:bool)
          n120 = case shown="True" w226 {
            tunnel: w224 -> [_ w233]
            tunnel: [w230 w231] -> w222
            tunnel: w223 -> [w230 w232]
            frame False {
            }
            frame True {
              n121 = Build Array (concatenate)(w232, w233) -> (w231:dbl[][])
            }
          }
          "SSD LOOP Counter" <- w219
        }
        "Steady-State Monitoring Variables 2" <- "Steady-State Monitoring Variables"
        "Steady-State Monitoring Variables 3" <- "Steady-State Monitoring Variables"
        "Steady-State Monitoring Variables 4" <- "Steady-State Monitoring Variables"
      }
      frame #4 {
        n122 = local read "Selected Data\nHeader Labels"() -> (w275:string[])
        n123 = Index Array(array=w274, index (col) #1="XY Graph1\nX-Variable", index (col) #2="XY Graph1\nY-Variable") -> (element #1=w283:dbl[], element #2=w292:dbl[])  [unwired: 2 in]
        n124 = Index Array(array=w274, index (col) #1="XY Graph2\nX-Variable 5", index (col) #2="XY Graph2\nY-Variable 5") -> (element #1=w298:dbl[], element #2=w287:dbl[])  [unwired: 2 in]
        n125 = Index Array(array=w274, index (col) #1="XY Graph2\nX-Variable 6", index (col) #2="XY Graph2\nY-Variable 6") -> (element #1=w282:dbl[], element #2=w279:dbl[])  [unwired: 2 in]
        n126 = Index Array(array=w274, index (col) #1="XY Graph2\nX-Variable 7", index (col) #2="XY Graph2\nY-Variable 7") -> (element #1=w280:dbl[], element #2=w269:dbl[])  [unwired: 2 in]
        n127 = Bundle(w283, w292) -> (→"XY Graph SS Filtered #1":cluster{dbl[], dbl[]})  [unwired: 1 in]
        n128 = Bundle(w298, w287) -> (→"XY Graph SS Filtered #2":cluster{dbl[], dbl[]})  [unwired: 1 in]
        n129 = Index Array(array=w275, index="XY Graph2\nY-Variable 6") -> (element=→"XY Graph1 Label 3":string)
        n130 = Bundle(w282, w279) -> (→"XY Graph SS Filtered #3":cluster{dbl[], dbl[]})  [unwired: 1 in]
        n131 = Index Array(array=w275, index="XY Graph2\nY-Variable 7") -> (element=→"XY Graph1 Label 4":string)
        n132 = Bundle(w280, w269) -> (→"XY Graph SS Filtered #4":cluster{dbl[], dbl[]})  [unwired: 1 in]
        n133 = Index Array(array=w275, index="XY Graph2\nY-Variable 5") -> (element=→"XY Graph1 Label 2":string)
        n134 = Index Array(array=w275, index="XY Graph1\nY-Variable") -> (element=→"XY Graph1 Label":string)
        n135 = call <vilib>:"Std Deviation and Variance.vi"("X"=w279) -> ("mean"=→"Mean Value Y5 2":dbl, "standard deviation"=→"St. Dev. Y5 2":dbl)  [unwired: 1 in, 1 out]
        n136 = call <vilib>:"Std Deviation and Variance.vi"("X"=w269) -> ("mean"=→"Mean Value Y5 3":dbl, "standard deviation"=→"St. Dev. Y5 3":dbl)  [unwired: 1 in, 1 out]
        n137 = call <vilib>:"Std Deviation and Variance.vi"("X"=w287) -> ("mean"=→"Mean Value Y5 6":dbl, "standard deviation"=→"St. Dev. Y5 6":dbl)  [unwired: 1 in, 1 out]
        n138 = call <vilib>:"Std Deviation and Variance.vi"("X"=w292) -> ("mean"=→"Mean Value Y":dbl, "standard deviation"=→"St. Dev. Y":dbl)  [unwired: 1 in, 1 out]
        n139 = Array Max & Min(array=w283) -> (max value=w286:dbl, min value=w285:dbl)  [unwired: 2 out]
        n140 = Subtract(x=w286, y=w285) -> (x-y=→"X-Variable RANGE":dbl)
        n141 = Array Size(array=w274) -> (size(s)=w293:i32[])
        "SS Filtered\nArray Size" <- w293
        n142 = Index Array(array=w293, index=0) -> (element=w264:i32)
      }
      frame #5 {
        n143 = Index Array(array=w307, index (col) #1="XY Graph2\nX-Variable 8", index (col) #2="XY Graph2\nY-Variable 8") -> (element #1=w320:dbl[], element #2=w319:dbl[])  [unwired: 2 in]
        n144 = Index Array(array=w307, index (col) #1="XY Graph2\nX-Variable 9", index (col) #2="XY Graph2\nY-Variable 9") -> (element #1=w312:dbl[], element #2=w311:dbl[])  [unwired: 2 in]
        n145 = local read "Selected Data\nHeader Labels"() -> (w310:string[])
        n146 = Index Array(array=w310, index="XY Graph2\nY-Variable 8") -> (element=→"XY Graph1 Label 5":string)
        n147 = Bundle(w320, w319) -> (→"XY Graph SS Filtered #5":cluster{dbl[], dbl[]})  [unwired: 1 in]
        n148 = Index Array(array=w310, index="XY Graph2\nY-Variable 9") -> (element=→"XY Graph1 Label 6":string)
        n149 = Bundle(w312, w311) -> (→"XY Graph SS Filtered #6":cluster{dbl[], dbl[]})  [unwired: 1 in]
        n150 = call <vilib>:"Std Deviation and Variance.vi"("X"=w319) -> ("mean"=→"Mean Value Y5 4":dbl, "standard deviation"=→"St. Dev. Y5 4":dbl)  [unwired: 1 in, 1 out]
        n151 = call <vilib>:"Std Deviation and Variance.vi"("X"=w311) -> ("mean"=→"Mean Value Y5 5":dbl, "standard deviation"=→"St. Dev. Y5 5":dbl)  [unwired: 1 in, 1 out]
      }
      frame #6 {
        n152 = flat-sequence {
          frame #0 {
            w321 = TRUE ("DONE")
            "DONE" <- w321
            "DONE 3" <- w321
            "DONE 4" <- w321
            "DONE 2" <- w321
          }
          frame #1 {
            n153 = Wait Until Next ms Multiple(millisecond multiple=u32 2000) -> ()  [unwired: 1 out]
          }
          frame #2 {
            n154 = while {
              stop <- "PAUSE?" continue-if-true
              n155 = Wait Until Next ms Multiple(millisecond multiple=u32 1000) -> ()  [unwired: 1 out]
            }
          }
        }
      }
      frame #7 {
        # "Current Filename"
        # "Save the Filtered Data."
        n156 = Path to Array of Strings(0:w329) -> (2:w328:string[])  [unwired: 1 out]
        n157 = Reverse 1D Array(array=w328) -> (reversed array=w327:string[])
        n158 = Index Array(array=w327, index=0) -> (element=w325:string)
        n159 = case shown="True" "SAVE the Conditional\nand SSD Filtered Data?" {
          tunnel: w331 -> [_ w352]
          tunnel: w329 -> [w334 w351]
          tunnel: "Output File" -> [w335 w347]
          tunnel: w325 -> [_ w342]
          frame False {
            n160 = call "Construct New Filename Ver013.vi"("Original Filename"=w334) -> ("New Filename with Path"=w336:path)  [unwired: 5 in, 4 out]
            n161 = Path To String(path=w335) -> (string=w338:string)
            n162 = Empty String/Path?(string/path=w338) -> (empty?=w337:bool)
            n163 = Select(t=w336, s=w337, f=w335) -> (s? t:f=w333:path)
            n164 = local write "Output File"(w333) -> ()
          }
          frame True {
            n165 = Number To Fractional String(number=w352) -> (F-format string=w343:string[][])  [unwired: 3 in]
            n166 = First Call?() -> (First Call?: T/F=w341:bool)
            n167 = for {
              tunnel: w343 -> [w363] mode=indexing
              tunnel: w342 -> [w361]
              tunnel: [w360] -> w340 mode=indexing
              # "Insert the data's filename into each row of SS Data."
              n168 = Insert Into Array(array=w363, index=0, new element=w361) -> (w360:string[])
            }
            n169 = case shown="False" w341 {
              tunnel: w340 -> [w353 w355]
              tunnel: [w353 w354] -> w339
              frame False {
              }
              frame True {
                n170 = local read "Selected Data\nHeader Labels"() -> (w358:string[])
                n171 = Insert Into Array(array=w358, index=0, new element="Filename" ("new element/subarray")) -> (w356:string[])
                n172 = Build Array (concatenate)(w356, w355) -> (w354:string[][])
              }
            }
            n173 = call "Construct New Filename Ver013.vi"("Original Filename"=w351) -> ("New Filename with Path"=w348:path)  [unwired: 5 in, 4 out]
            n174 = Path To String(path=w347) -> (string=w350:string)
            n175 = Empty String/Path?(string/path=w350) -> (empty?=w349:bool)
            n176 = Select(t=w348, s=w349, f=w347) -> (s? t:f=w344:path)
            n177 = local write "Output File"(w344) -> ()
            n178 = call-poly <vilib>:"Write Delimited Spreadsheet.vi"("file path (dialog if empty)"=w344, "2D data"=w339, "append to file? (new file:F)"="Append to File (T) or\nMake NEW FILE (F)?") -> ("error out"=→"Write Output error out":errorcluster)  [unwired: 11 in, 1 out]
          }
        }
      }
      frame #8 {
        w371 = FALSE ("Loop1")
        n179 = Get Date/Time In Seconds() -> (seconds since 1Jan1904=w376:timestamp)
        n180 = Subtract(x=w376, y=w375) -> (x-y=w374:dbl)
        n181 = Multiply(x=1000.0, y=w374) -> (x*y=→"Time to Execute\nSCAN (millisecond)":dbl)
        n182 = local write "Loop1"(w371) -> ()
        n183 = local write "Loop2"(w371) -> ()
        n184 = To Double Precision Float(number=w367) -> (double precision float=w366:dbl)
        n185 = To Double Precision Float(number=w365) -> (double precision float=w364:dbl)
        n186 = Divide(x=w366, y=w364) -> (x/y=w368:dbl)
        n187 = Multiply(x=w368, y=100.0) -> (x*y=→"% Retained":dbl)
      }
    }
  }
